vi "camera config.vi"() -> ()   [LabVIEW 2015]
panel:
  in  "Cancel Button":bool
  out "Image Out":T1(plugin-control)
  in  "OK Button":bool
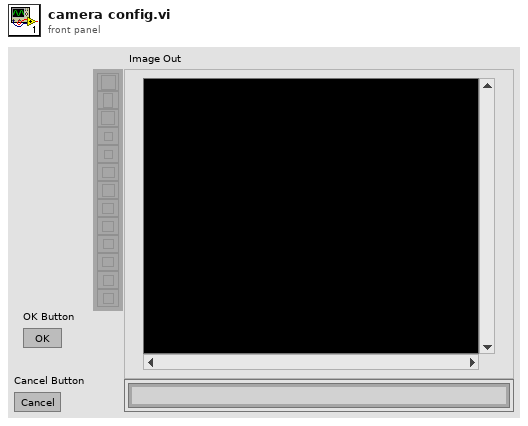
[diagram p1: front panel]
types:
  T1 = typedef "IMAQ Image.ctl" = refnum<image>
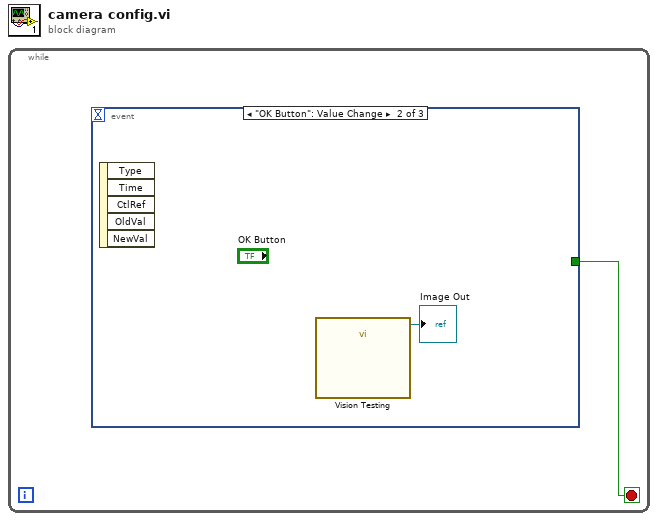
[diagram p0: block diagram]
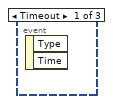
[diagram p2: hidden frame]
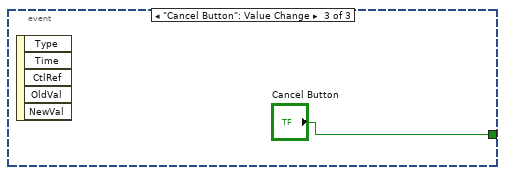
[diagram p3: hidden frame]
diagram:
  n1 = while {
    stop <- w1 stop-if-true
    n2 = event shown="[1] \"OK Button\": Value Change" {
      selector: _ -> [_ _ _]
      dyn-events: _ -> [_ _ _]
      timeout: _ -> [_ _ _]
      tunnel: [_ _ "Cancel Button"] -> w1
      event Timeout {
        n3 = event-data() -> ()  [unwired: 1 in, 2 out]
      }
      event "OK Button": Value Change {
        n4 = event-data() -> ()  [unwired: 1 in, 5 out]
        n5 = call "Vision Testing.vi"() -> ("Image Out"=→"Image Out":T1)  [unwired: 26 in, 1 out]
      }
      event "Cancel Button": Value Change {
        n6 = event-data() -> ()  [unwired: 1 in, 5 out]
      }
    }
  }
